vi "Smoke Test.vi"() -> ()   [LabVIEW 2020]
uses:
  <vilib>/gpm_packages/@cs/user-manager/Source/User Configuration Manager/User Configuration Manager.lvclass
  C:/Program Files/National Instruments/LabVIEW 2020/vi.lib/gpm_packages/@cs/user-manager/Source/iUser Configuration Manager/iUser Configuration Manager.lvclass
  <vilib>/gpm_packages/@cs/user-manager/Source/SHA-1 Encryption/SHA-1.lvclass
  C:/Program Files/National Instruments/LabVIEW 2020/vi.lib/gpm_packages/@cs/user-manager/Source/iEncryption/iEncryption.lvclass
  <vilib>/gpm_packages/@cs/user-manager/Source/User Configuration Manager Ref/By Ref.lvlib
panel:
  out "logical AND":bool
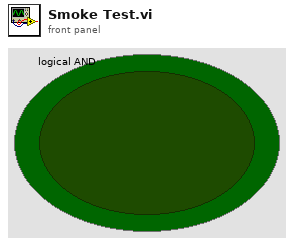
[diagram p1: front panel]
types:
  T1 = cluster{"Attribute Name":string, "Attribute Value":variant}
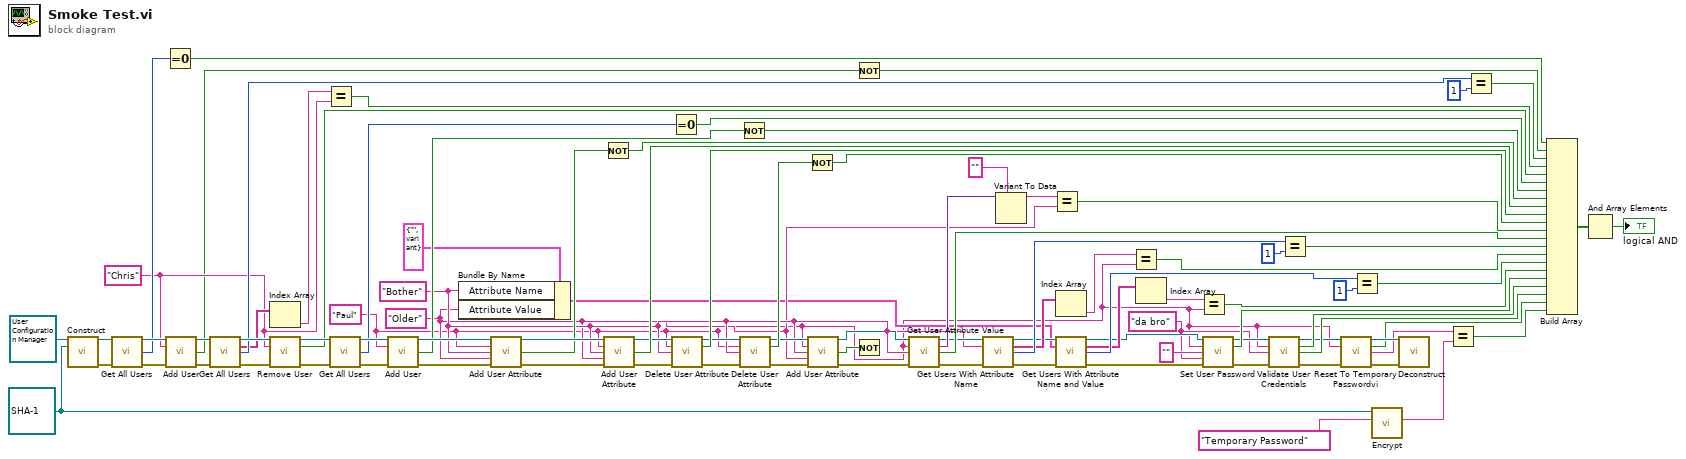
[diagram p0: block diagram]
diagram:
  w3 = refnum<class "SHA-1.lvclass"> refnum ("User Configuration Manager.lvlib:SHA-1.lvclass")
  w15 = "da bro" ("New Password")
  w26 = "Older" ("Attribute Name")
  w32 = "Bother" ("Attribute Name")
  w7 = "Paul" ("Username")
  w78 = "Chris" ("Username")
  n1 = call <vilib>:"Construct.vi"("iUser Configuration Manager in"=refnum<class "User Configuration Manager.lvclass"> refnum ("User Configuration Manager.lvlib:User Configuration Manager"), "Encryption Type"=w3) -> ("dup iUser Configuration Manager DVR"=w95:refnum<data-value>, "error out"=w94:errorcluster)  [unwired: 12 in]
  n2 = call <vilib>:"Get All Users.vi"("iUser Configuration Manager DVR"=w95, "error in"=w94) -> ("dup iUser Configuration Manager DVR"=w93:refnum<data-value>, "Number of Users Found"=w83:u32, "error out"=w92:errorcluster)  [unwired: 10 in, 1 out]
  n3 = Equal To 0?(x=w83) -> (x = 0?=w71:bool)
  n4 = call <vilib>:"Add User.vi"("iUser Configuration Manager DVR"=w93, "Username"=w78, "error in"=w92) -> ("dup iUser Configuration Manager DVR"=w91:refnum<data-value>, "Replaced"=w70:bool, "error out"=w90:errorcluster)  [unwired: 10 in]
  n5 = call <vilib>:"Get All Users.vi"("iUser Configuration Manager DVR"=w91, "error in"=w90) -> ("dup iUser Configuration Manager DVR"=w89:refnum<data-value>, "Users"=w80:string[], "Number of Users Found"=w82:u32, "error out"=w88:errorcluster)  [unwired: 10 in]
  n6 = Index Array(array=w80) -> (element=w79:string)  [unwired: 1 in]
  n7 = call <vilib>:"Remove User.vi"("iUser Configuration Manager DVR"=w89, "Username"=w78, "error in"=w88) -> ("dup iUser Configuration Manager DVR"=w87:refnum<data-value>, "Found"=w66:bool, "error out"=w86:errorcluster)  [unwired: 10 in]
  n8 = Equal?(x=w79, y=w78) -> (x = y?=w67:bool)
  n9 = call <vilib>:"Get All Users.vi"("iUser Configuration Manager DVR"=w87, "error in"=w86) -> ("dup iUser Configuration Manager DVR"=w85:refnum<data-value>, "Number of Users Found"=w77:u32, "error out"=w84:errorcluster)  [unwired: 10 in, 1 out]
  n10 = call <vilib>:"Add User.vi"("iUser Configuration Manager DVR"=w85, "Username"=w7, "error in"=w84) -> ("dup iUser Configuration Manager DVR"=w76:refnum<data-value>, "Replaced"=w64:bool, "error out"=w75:errorcluster)  [unwired: 10 in]
  n11 = Bundle By Name(cluster=T1 {"Attribute Name"="", "Attribute Value"=variant} ("Query"), "Attribute Name"=w32, "Attribute Value"=w26) -> (w23:T1)
  n12 = call <vilib>:"Add User Attribute.vi"("iUser Configuration Manager DVR"=w76, "Username"=w7, "Attribute Name"=w32, "Attribute Value"=w26, "error in"=w75) -> ("dup iUser Configuration Manager DVR"=w74:refnum<data-value>, "Replaced"=w72:bool, "error out"=w73:errorcluster)  [unwired: 8 in]
  n13 = Not(x=w72) -> (.not. x?=w62:bool)
  n14 = call <vilib>:"Add User Attribute.vi"("iUser Configuration Manager DVR"=w74, "Username"=w7, "Attribute Name"=w32, "Attribute Value"=w26, "error in"=w73) -> ("dup iUser Configuration Manager DVR"=w59:refnum<data-value>, "Replaced"=w61:bool, "error out"=w58:errorcluster)  [unwired: 8 in]
  n15 = Equal To 0?(x=w77) -> (x = 0?=w65:bool)
  n16 = call <vilib>:"Delete User Attribute.vi"("iUser Configuration Manager DVR"=w59, "Username"=w7, "Attribute Name"=w32, "error in"=w58) -> ("dup iUser Configuration Manager DVR"=w56:refnum<data-value>, "Found"=w57:bool, "error out"=w55:errorcluster)  [unwired: 9 in]
  n17 = Not(x=w64) -> (.not. x?=w63:bool)
  n18 = call <vilib>:"Delete User Attribute.vi"("iUser Configuration Manager DVR"=w56, "Username"=w7, "Attribute Name"=w32, "error in"=w55) -> ("dup iUser Configuration Manager DVR"=w52:refnum<data-value>, "Found"=w54:bool, "error out"=w51:errorcluster)  [unwired: 9 in]
  n19 = Not(x=w54) -> (.not. x?=w53:bool)
  n20 = call <vilib>:"Add User Attribute.vi"("iUser Configuration Manager DVR"=w52, "Username"=w7, "Attribute Name"=w32, "Attribute Value"=w26, "error in"=w51) -> ("dup iUser Configuration Manager DVR"=w50:refnum<data-value>, "Replaced"=w49:bool, "error out"=w48:errorcluster)  [unwired: 8 in]
  n21 = Not(x=w70) -> (.not. x?=w69:bool)
  n22 = Not(x=w49) -> ()  [unwired: 1 out]
  n23 = call <vilib>:"Get User Attribute Value.vi"("iUser Configuration Manager DVR"=w50, "Username"=w7, "Attribute Name"=w32, "error in"=w48) -> ("dup iUser Configuration Manager DVR"=w42:refnum<data-value>, "Attribute Value"=w47:variant, "Found"=w43:bool, "error out"=w41:errorcluster)  [unwired: 8 in]
  n24 = call <vilib>:"Get Users With Attribute Name.vi"("iUser Configuration Manager DVR"=w42, "Attribute Name"=w32, "error in"=w41) -> ("dup iUser Configuration Manager DVR"=w34:refnum<data-value>, "Users"=w37:string[], "Number of Users Found"=w39:u32, "error out"=w33:errorcluster)  [unwired: 9 in]
  n25 = Variant To Data(type="" ("Attribute Name"), Variant=w47) -> (data=w45:string)  [unwired: 1 in, 1 out]
  n26 = Equal?(x=w45, y=w26) -> (x = y?=w44:bool)
  n27 = Index Array(array=w37) -> (element=w38:string)  [unwired: 1 in]
  n28 = call <vilib>:"Get Users With Attribute Name and Value.vi"("iUser Configuration Manager DVR"=w34, "Query"=w23, "error in"=w33) -> ("dup iUser Configuration Manager DVR"=w20:refnum<data-value>, "Users"=w27:string[], "Number of Users Found"=w30:u32, "error out"=w19:errorcluster)  [unwired: 9 in]
  n29 = Equal?(x=w38, y=w7) -> (x = y?=w35:bool)
  n30 = Index Array(array=w27) -> (element=w28:string)  [unwired: 1 in]
  n31 = Equal?(x=w28, y=w7) -> (x = y?=w25:bool)
  n32 = call <vilib>:"Set User Password.vi"("iUser Configuration Manager DVR"=w20, "Username"=w7, "Current Password"="", "New Password"=w15, "error in"=w19) -> ("dup iUser Configuration Manager DVR"=w16:refnum<data-value>, "Found"=w17:bool, "error out"=w14:errorcluster)  [unwired: 8 in]
  n33 = call <vilib>:"Validate User Credentials.vi"("iUser Configuration Manager DVR"=w16, "Username"=w7, "Password"=w15, "error in"=w14) -> ("dup iUser Configuration Manager DVR"=w11:refnum<data-value>, "User Found"=w13:bool, "Verified"=w12:bool, "error out"=w9:errorcluster)  [unwired: 7 in, 1 out]
  n34 = Equal?(x=w39, y=u32 1) -> (x = y?=w36:bool)
  n35 = call <vilib>:"Reset To Temporary Passwordvi.vi"("iUser Configuration Manager DVR"=w11, "Username"=w7, "error in"=w9) -> ("dup iUser Configuration Manager DVR"=w10:refnum<data-value>, "User Found"=w6:bool, "Temporary Password"=w5:string, "error out"=w8:errorcluster)  [unwired: 9 in]
  n36 = Equal?(x=w30, y=u32 1) -> (x = y?=w29:bool)
  n37 = call-dynamic "Encrypt.vi"("String"="Temporary Password" ("y"), "SHA-1 in"=w3) -> ("Encrypted String"=w1:string)  [unwired: 9 in]
  n38 = call <vilib>:"Deconstruct.vi"("iUser Configuration Manager DVR"=w10, "Error In"=w8) -> ()  [unwired: 13 in, 1 out]
  n39 = Equal?(x=w5, y=w1) -> (x = y?=w4:bool)
  n40 = Equal?(x=w82, y=u32 1) -> (x = y?=w68:bool)
  n41 = Build Array(w71, w69, w68, w67, w66, w65, w63, w62, w61, w57, w53, w44, w43, w36, w35, w29, w25, w17, w13, w12, w6, w4) -> (w22:bool[])
  n42 = And Array Elements(Boolean array=w22) -> (logical AND=→"logical AND":bool)
